vi "Insert Halt.vi"(6 "Insertion Index":i32=-1, 7 "Parent ID":string, 8 "error in (no error)":errorcluster, 9 "Unique ID":string, 10 "Name":string, 11 "Test Executive Ref":refnum<data-value>) -> (0 "error out":errorcluster, 1 "Replaced?":bool, 3 "Test Executive Ref out":refnum<data-value>, 5 "Unique ID out":string)   [LabVIEW 2020, in "Test Executive.lvlib" / "TestExecutive Ref.lvclass"]
uses:
  <vilib>/gpm_packages/@cs/test-executive/Source/Test Executive/TestExecutive Ref/TestExecutive Ref.lvclass
  <vilib>/gpm_packages/@cs/test-executive/Source/Test Executive/ITestExecutive/ITest Executive.lvclass
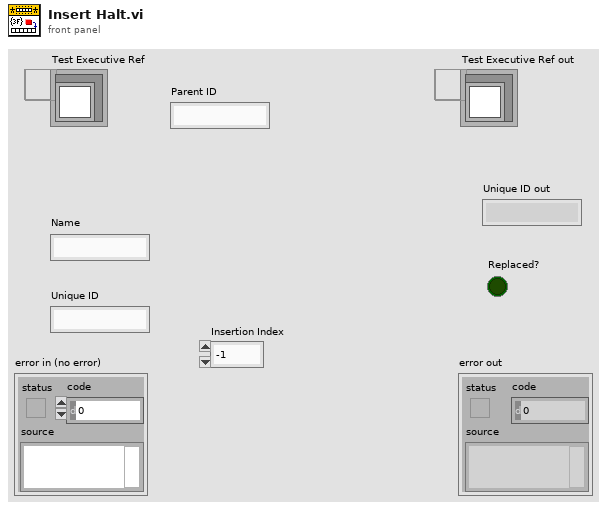
[diagram p1: front panel]
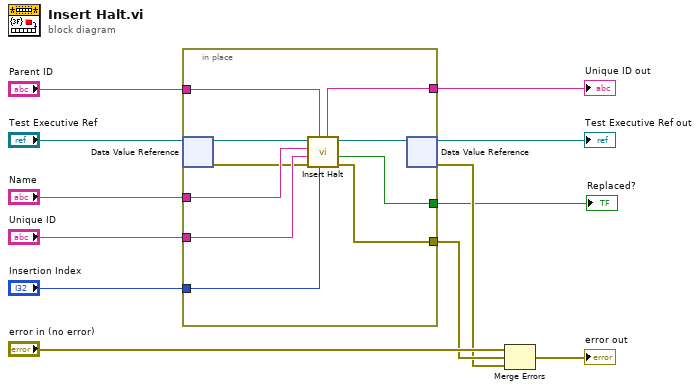
[diagram p0: block diagram]
diagram:
  n1 = in-place {
    in-place-border: "Parent ID" -> [w22]
    in-place-border: "Name" -> [w18]
    in-place-border: "Unique ID" -> [w17]
    in-place-border: "Insertion Index" -> [w13]
    in-place-border: [w21] -> w6
    in-place-border: [w15] -> w4
    in-place-border: [w14] -> w1
    n2 = in-place-dvr #1("Test Executive Ref") -> (w20:refnum<class "ITest Executive.lvclass">, w16:errorcluster)
    n3 = call-dynamic "Insert Halt.vi"("Insertion Index"=w13, "Parent ID"=w22, "error in (no error)"=w16, "Unique ID"=w17, "Name"=w18, "ITest Executive in"=w20) -> ("error out"=w15:errorcluster, "Replaced?"=w14:bool, "ITest Executive out"=w19:refnum<class "ITest Executive.lvclass">, "Unique ID out"=w21:string)  [unwired: 2 in]
    n4 = in-place-dvr #1(w19) -> (→"Test Executive Ref out":refnum<data-value>, w3:errorcluster)
  }
  "Unique ID out" <- w6
  "Replaced?" <- w1
  n5 = Merge Errors("error in (no error)", w4, w3) -> (→"error out":errorcluster)
